vi "Get Object.vi"(8 "error in":errorcluster, 9 "Sub-Index":i16=-1, 10 "Index":u16 format="%04x", 11 "Sorted Object Dictionary in":refnum<class "Sorted Object Dictionary.lvclass">) -> (0 "error out":errorcluster, 1 "OD Entry":refnum<class "OD Entry.lvclass">, 2 "Found?":bool, 3 "Sorted Object Dictionary out":refnum<class "Sorted Object Dictionary.lvclass">)   [LabVIEW 2019, in "Electronic Datasheet.lvlib" / "Sorted Object Dictionary.lvclass"]
uses:
  Sorted Object Dictionary.lvclass
  OD Entry/OD Entry.lvclass
  Sorted Object Dictionary.lvclass/Sorted Object Dictionary.ctl
  OD Sub-Entry/OD Sub-Entry.lvclass
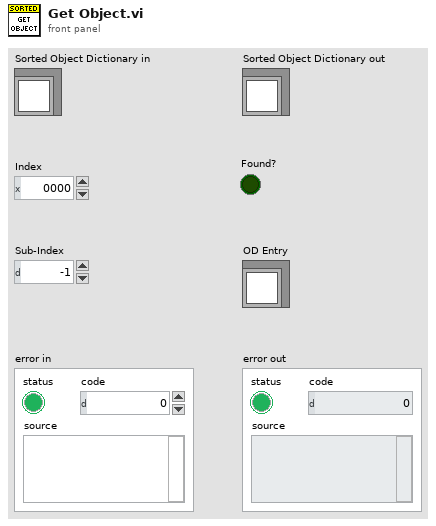
[diagram p1: front panel]
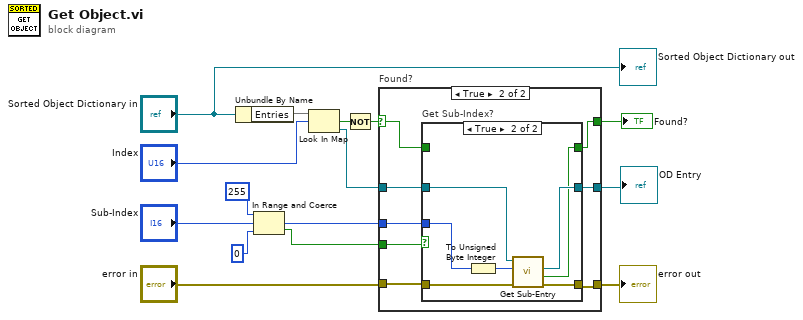
[diagram p0: block diagram]
diagram:
  n1 = Unbundle By Name("Sorted Object Dictionary in") -> ("Entries"=w10:map{u16, refnum<class "OD Entry.lvclass">})
  n2 = In Range and Coerce(upper limit=i16 255, x="Sub-Index", lower limit=i16 0) -> (coerced(x)=w5:i16, In Range?=w2:bool)
  n3 = Look In Map(map=w10, key="Index") -> (key not found?=w9:bool, value=w8:refnum<class "OD Entry.lvclass">)  [unwired: 1 in]
  n4 = Not(x=w9) -> (.not. x?=w7:bool)
  n5 = case "Found?" shown="True" w7 {
    selector: w7 -> [w17 w19]
    tunnel: [w17 w20] -> w15
    tunnel: w8 -> [w16 w22]
    tunnel: [w16 w21] -> w14
    tunnel: "error in" -> [w18 w26]
    tunnel: [w18 w25] -> w13
    tunnel: w2 -> [_ w24]
    tunnel: w5 -> [_ w23]
    frame False {
    }
    frame True {
      n6 = case "Get Sub-Index?" shown="True" w24 {
        tunnel: w26 -> [w29 w34]
        tunnel: [w29 w33] -> w25
        tunnel: w23 -> [_ w36]
        tunnel: w22 -> [w28 w35]
        tunnel: [w28 w32] -> w21
        tunnel: [w27 w31] -> w20
        tunnel: w19 -> [w27 _]
        frame False {
        }
        frame True {
          n7 = To Unsigned Byte Integer(number=w36) -> (unsigned 8bit integer=w30:u8)
          n8 = call "Get Sub-Entry.vi"("Error In"=w34, "Sub-Index"=w30, "reference in"=w35) -> ("Error Out"=w33:errorcluster, "Found?"=w31:bool, "OD Sub-Entry"=w32:refnum<class "OD Sub-Entry.lvclass">)  [unwired: 5 in, 1 out]
        }
      }
    }
  }
  "OD Entry" <- w14
  "Found?" <- w15
  "error out" <- w13
  "Sorted Object Dictionary out" <- "Sorted Object Dictionary in"
